vi "controlMove.vi"(7 "Set":bool, 8 "error in":errorcluster, 9 "control move in":bool=TRUE, 10 "axis in":u8, 11 "connection ID":refnum<k5>) -> (0 "error out":errorcluster, 1 "controll move out":bool=TRUE, 2 "axis out":u8, 3 "connection ID":refnum<k5>)   [LabVIEW 2016]
doc: "This function retrieves or sets the approach of the selected axis positioner to the target position."
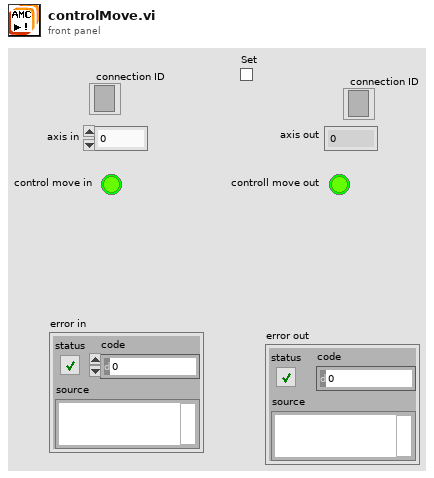
[diagram p1: front panel]
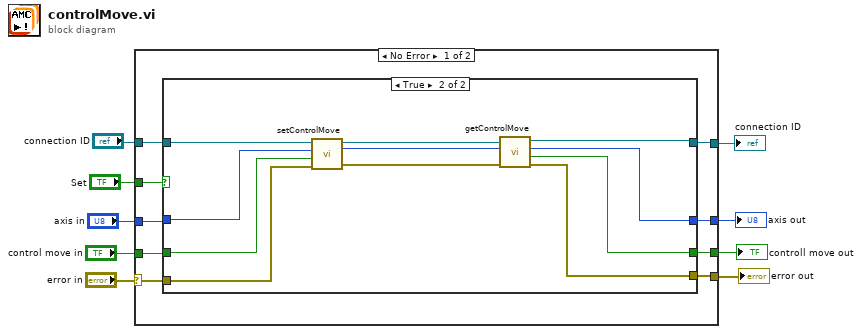
[diagram p0: block diagram]
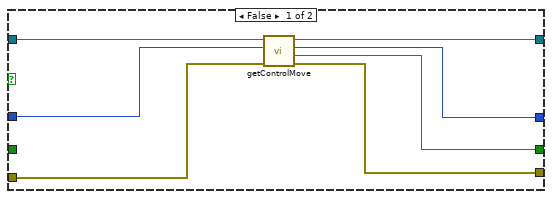
[diagram p2: hidden frame]
diagram:
  n1 = case shown="No Error" "error in" {
    selector: "error in" -> [w10 w40]
    tunnel: "axis in" -> [w16 w38]
    tunnel: [w11 w40] -> w8
    tunnel: [w13 w38] -> w7
    tunnel: "Set" -> [w17 _]
    tunnel: [w12 w39] -> w5
    tunnel: "control move in" -> [w15 w39]
    tunnel: [w14 w37] -> w3
    tunnel: "connection ID" -> [w18 w37]
    frame No Error {
      n2 = case shown="True" w17 {
        tunnel: [w24 w31] -> w14
        tunnel: w18 -> [w25 w35]
        tunnel: w16 -> [w20 w36]
        tunnel: [w19 w29] -> w13
        tunnel: [w22 w28] -> w11
        tunnel: [w21 w26] -> w12
        tunnel: w15 -> [_ w33]
        tunnel: w10 -> [w23 w34]
        frame False {
          n3 = call "getControlMove.vi"("error in"=w23, "axis"=w20, "connection ID"=w25) -> ("error out"=w22:errorcluster, "enable"=w21:bool, "axis_out"=w19:i32, "connection ID"=w24:refnum<k5>)  [unwired: 5 in]
        }
        frame True {
          n4 = call "setControlMove.vi"("error in"=w34, "enable"=w33, "axis"=w36, "connection ID"=w35) -> ("error out"=w27:errorcluster, "axis_out"=w30:i32, "connection ID"=w32:refnum<k5>)  [unwired: 5 in]
          n5 = call "getControlMove.vi"("error in"=w27, "axis"=w30, "connection ID"=w32) -> ("error out"=w28:errorcluster, "enable"=w26:bool, "axis_out"=w29:i32, "connection ID"=w31:refnum<k5>)  [unwired: 5 in]
        }
      }
    }
    frame Error {
    }
  }
  "error out" <- w8
  "axis out" <- w7
  "controll move out" <- w5
  "connection ID" <- w3
